vi "Update_File_Name.vi"(3 "Number of Channels":i32, 4 "New File":bool, 5 "File Path IN":path) -> (0 "Text Image Data Path":path, 1 "File References":path[](array[path]), 2 "File Path OUT":path)   [LabVIEW 2014]
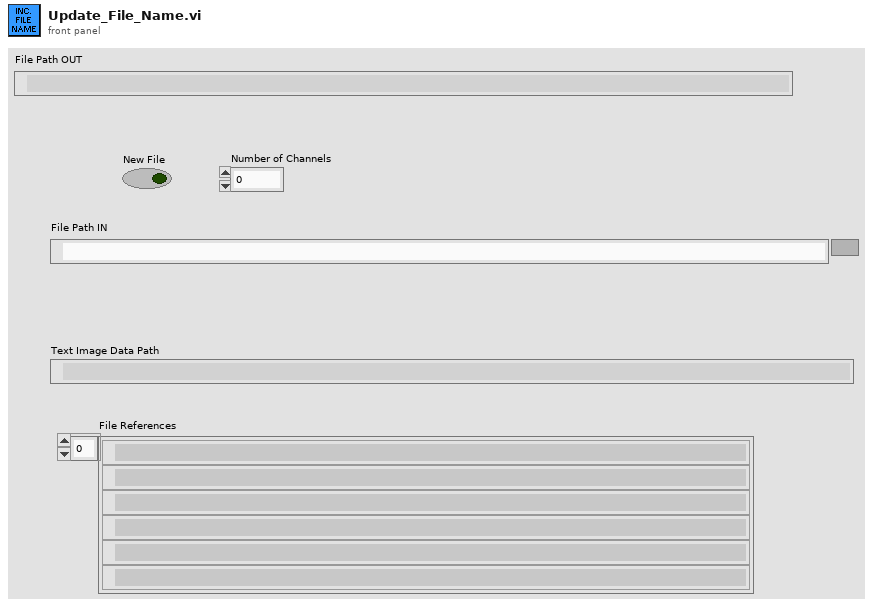
[diagram p1: front panel]
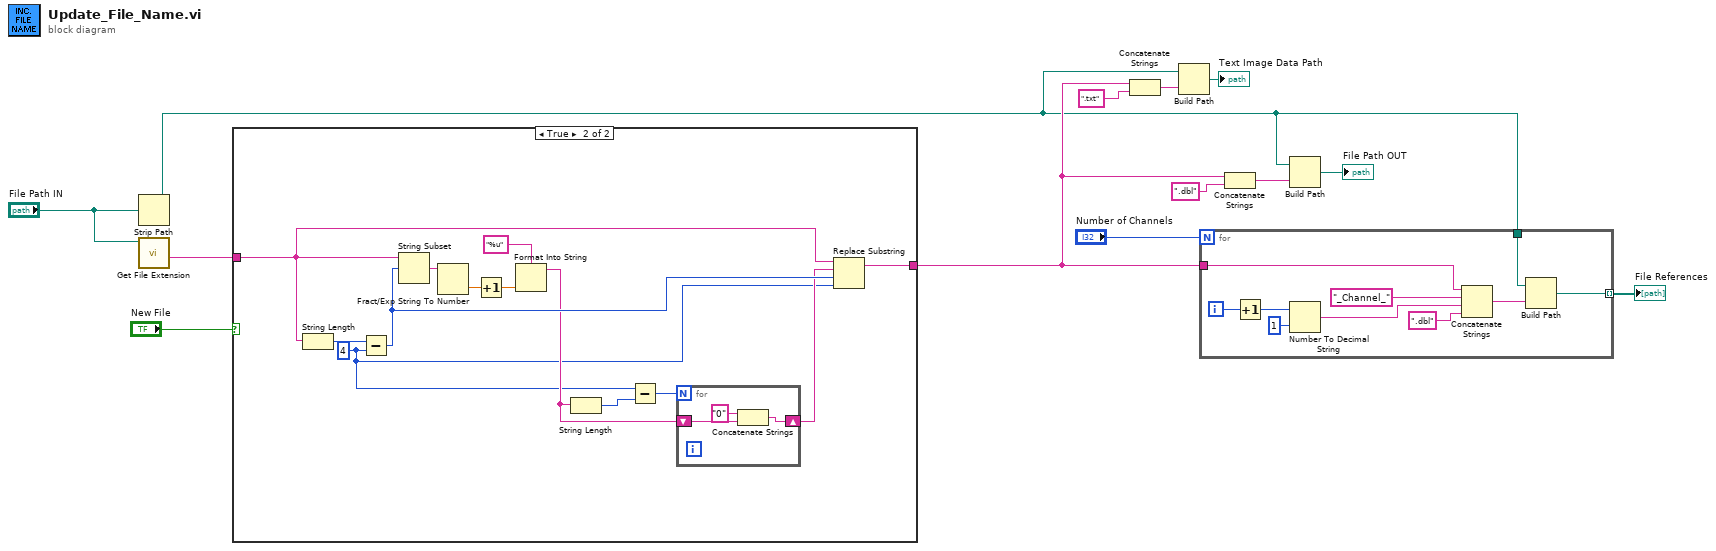
[diagram p0: block diagram]
diagram:
  n1 = Strip Path(path="File Path IN") -> (stripped path=w2:path)  [unwired: 1 out]
  n2 = call <vilib>:"Get File Extension.vi"("file"="File Path IN") -> ("filename without extension"=w13:string)  [unwired: 7 in, 3 out]
  n3 = case shown="True" "New File" {
    tunnel: w13 -> [w14 w23]
    tunnel: [w14 w15] -> w4
    frame False {
    }
    frame True {
      w16 = 4 ("y")
      n4 = String Length(string=w23) -> (length=w27:i32)
      n5 = Subtract(x=w27, y=w16) -> (x-y=w22:i32)
      n6 = String Subset(string=w23, offset (0)=w22) -> (substring=w26:string)  [unwired: 1 in]
      n7 = Fract/Exp String To Number(string=w26) -> (number=w25:dbl)  [unwired: 3 in, 1 out]
      n8 = Increment(x=w25) -> (x+1=w24:dbl)
      n9 = Format Into String(format string="%u", w24) -> (resulting string=w19:string)  [unwired: 2 in, 1 out]
      n10 = String Length(string=w19) -> (length=w17:i32)
      n11 = Subtract(x=w16, y=w17) -> (x-y=w20:i32)
      n12 = for {
        N: w20 -> [_]
        shift-right: [w29] -> w18
        shift-left: w19 -> [w30]
        n13 = Concatenate Strings("0" ("string"), w30) -> (w29:string)
      }
      n14 = Replace Substring(2:w16, 3:w22, 4:w18, 5:w23) -> (1:w15:string)  [unwired: 1 out]
    }
  }
  n15 = Concatenate Strings(w4, ".txt" ("string")) -> (w10:string)
  n16 = Build Path(base path=w2, name or relative path=w10) -> (appended path=→"Text Image Data Path":path)
  n17 = for {
    N: "Number of Channels" -> [_]
    tunnel: w4 -> [w37]
    tunnel: w2 -> [w33]
    tunnel: [w31] -> w6 mode=indexing
    i -> [w40]
    n18 = Increment(x=w40) -> (x+1=w35:i32)
    n19 = Number To Decimal String(number=w35, width (-)=i16 1) -> (decimal integer string=w34:string)
    n20 = Concatenate Strings(w37, "_Channel_" ("string"), w34, ".dbl" ("string")) -> (w32:string)
    n21 = Build Path(base path=w33, name or relative path=w32) -> (appended path=w31:path)
  }
  "File References" <- w6
  n22 = Concatenate Strings(w4, ".dbl" ("string")) -> (w3:string)
  n23 = Build Path(base path=w2, name or relative path=w3) -> (appended path=→"File Path OUT":path)
